vi "Counter_DetectCntrEvent.vi"(3 "error in (no error)":errorcluster, 4 "status":bool, 5 "Task ID":u32) -> (0 "error out":errorcluster, 1 "interrupt?":bool, 2 "Task out ID":u32)   [LabVIEW 2015]
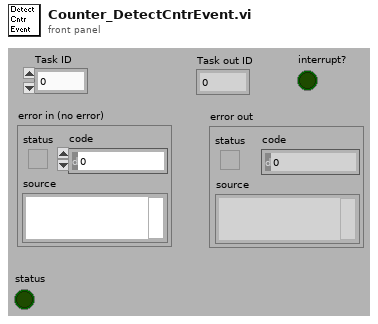
[diagram p1: front panel]
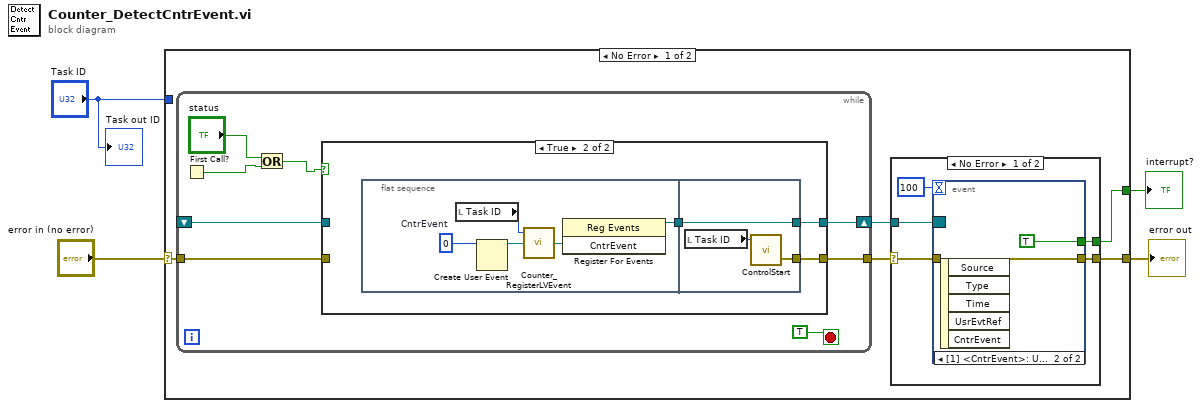
[diagram p0: block diagram]
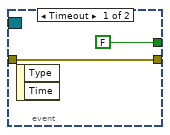
[diagram p2: hidden frame]
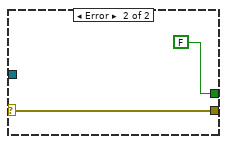
[diagram p3: hidden frame]
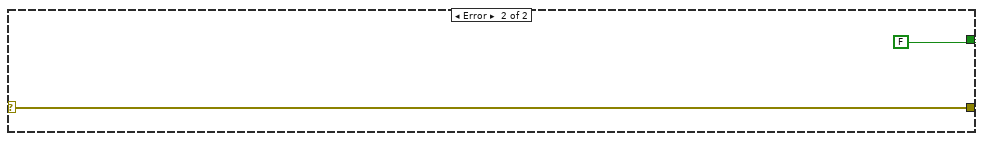
[diagram p5: hidden frame]
diagram:
  n1 = case shown="No Error" "error in (no error)" {
    selector: "error in (no error)" -> [w5 w42]
    tunnel: "Task ID" -> [_ _]
    tunnel: [w9 FALSE] -> w3
    tunnel: [w8 w42] -> w2
    frame No Error {
      n2 = while {
        shift-right: [w27] -> w7
        shift-left: _ -> [w26]
        tunnel: [w25] -> w6
        tunnel: w5 -> [w24]
        stop <- TRUE stop-if-true
        n3 = First Call?() -> (First Call?: T/F=w22:bool)
        n4 = Or(x="status", y=w22) -> (x .or. y?=w21:bool)
        n5 = case shown="True" w21 {
          tunnel: [w30 w32] -> w27
          tunnel: w26 -> [w30 _]
          tunnel: [w29 w31] -> w25
          tunnel: w24 -> [w29 _]
          frame False {
          }
          frame True {
            n6 = flat-sequence {
              tunnel: [w34] -> w33
              tunnel: [w40] -> w32
              tunnel: w33 -> [w40]
              tunnel: [w39] -> w31
              frame #0 {
                w38 = 0  # CntrEvent
                n7 = local read "Task ID"() -> (w37:u32)
                n8 = Create User Event(user event datatype=w38) -> (user event=w36:refnum<user-event>)  [unwired: 1 in, 1 out]
                n9 = call "Counter_RegisterLVEvent.vi"("CntrEvent"=w36, "Task ID"=w37) -> ("CntrEvent"=w35:refnum<user-event>)  [unwired: 1 in, 2 out]
                n10 = register-events(w35) -> (reference out=w34:refnum<event-registration>)  [unwired: 2 in, 1 out]
              }
              frame #1 {
                n11 = local read "Task ID"() -> (w41:u32)
                n12 = call "ControlStart.vi"("Task ID"=w41) -> ("error out"=w39:errorcluster)  [unwired: 1 in, 2 out]
              }
            }
          }
        }
      }
      n13 = case shown="No Error" w6 {
        selector: w6 -> [w11 w19]
        tunnel: w7 -> [w14 _]
        tunnel: [w13 FALSE] -> w9
        tunnel: [w10 w19] -> w8
        frame No Error {
          n14 = event shown="[1] <CntrEvent>: User Event" {
            selector: w14 -> [_ _]
            dyn-events: _ -> [_ _]
            timeout: 100 -> [_ _]
            tunnel: [FALSE TRUE] -> w13
            tunnel: w11 -> [w15 w17]
            tunnel: [w15 w17] -> w10
            event Timeout {
              n15 = event-data() -> ()  [unwired: 3 out]
            }
            event User Event {
              n16 = event-data() -> ()  [unwired: 6 out]
            }
          }
        }
        frame Error {
        }
      }
    }
    frame Error {
    }
  }
  "error out" <- w2
  "interrupt?" <- w3
  "Task out ID" <- "Task ID"
